vi "loadorsave_Option.vi"(6 "save?":bool, 8 "error in":errorcluster, 10 "Caldata in":T1={"分辨率"="", "Fps"=0, "工单号"="", "操作人"="", "增益模式"=enum."高低增益切换", "黑体设定温度1"=0.0, "温差范围1"=0.0, "出图到测温等待时间"=0.0, "调焦数值min"=0, "盲元阈值"=0.0, "盲元采样帧数"=0, "调焦数值min2"=0, "黑体设定温度2"=0.0, "温差范围2"=0.0, "ID选择"=enum."新ID", "快门时间间隔设置"={"快门第一次延时时间"=200, "快门第二次延时时间"=200, "切换增益后快门第一次延时时间"=200, "切换增益后快门第二次延时时间"=200}, "产品名"="Tiny1-C", "镜头"="02011X", "测温功能"="WR", "产品料号"="", "打印机VISA"="", "焦距选择"=enum."Radio Selection 1", "工位"="0001", "服务器保存地址"=path ""}, 11 "Path in":path) -> (0 "error out":errorcluster, 2 "Caldata out":T1={"分辨率"="", "Fps"=0, "工单号"="", "操作人"="", "增益模式"=enum."高低增益切换", "黑体设定温度1"=0.0, "温差范围1"=0.0, "出图到测温等待时间"=0.0, "调焦数值min"=0, "盲元阈值"=0.0, "盲元采样帧数"=0, "调焦数值min2"=0, "黑体设定温度2"=0.0, "温差范围2"=0.0, "ID选择"=enum."新ID", "快门时间间隔设置"={"快门第一次延时时间"=200, "快门第二次延时时间"=200, "切换增益后快门第一次延时时间"=200, "切换增益后快门第二次延时时间"=200}, "产品名"="Tiny1-C", "镜头"="02011X", "测温功能"="WR", "产品料号"="", "打印机VISA"="", "焦距选择"=enum."Radio Selection 1", "工位"="0001", "服务器保存地址"=path ""}, 3 "Path out":path)   [LabVIEW 2016]
uses:
  Ctl/Option.ctl
panel:
  out "Caldata ctl":T1={"分辨率"="", "Fps"=0, "工单号"="", "操作人"="", "增益模式"=enum."高低增益切换", "黑体设定温度1"=0.0, "温差范围1"=0.0, "出图到测温等待时间"=0.0, "调焦数值min"=0, "盲元阈值"=0.0, "盲元采样帧数"=0, "调焦数值min2"=0, "黑体设定温度2"=0.0, "温差范围2"=0.0, "ID选择"=enum."新ID", "快门时间间隔设置"={"快门第一次延时时间"=200, "快门第二次延时时间"=200, "切换增益后快门第一次延时时间"=200, "切换增益后快门第二次延时时间"=200}, "产品名"="Tiny1-C", "镜头"="02011X", "测温功能"="WR", "产品料号"="", "打印机VISA"="", "焦距选择"=enum."Radio Selection 1", "工位"="0001", "服务器保存地址"=path ""}
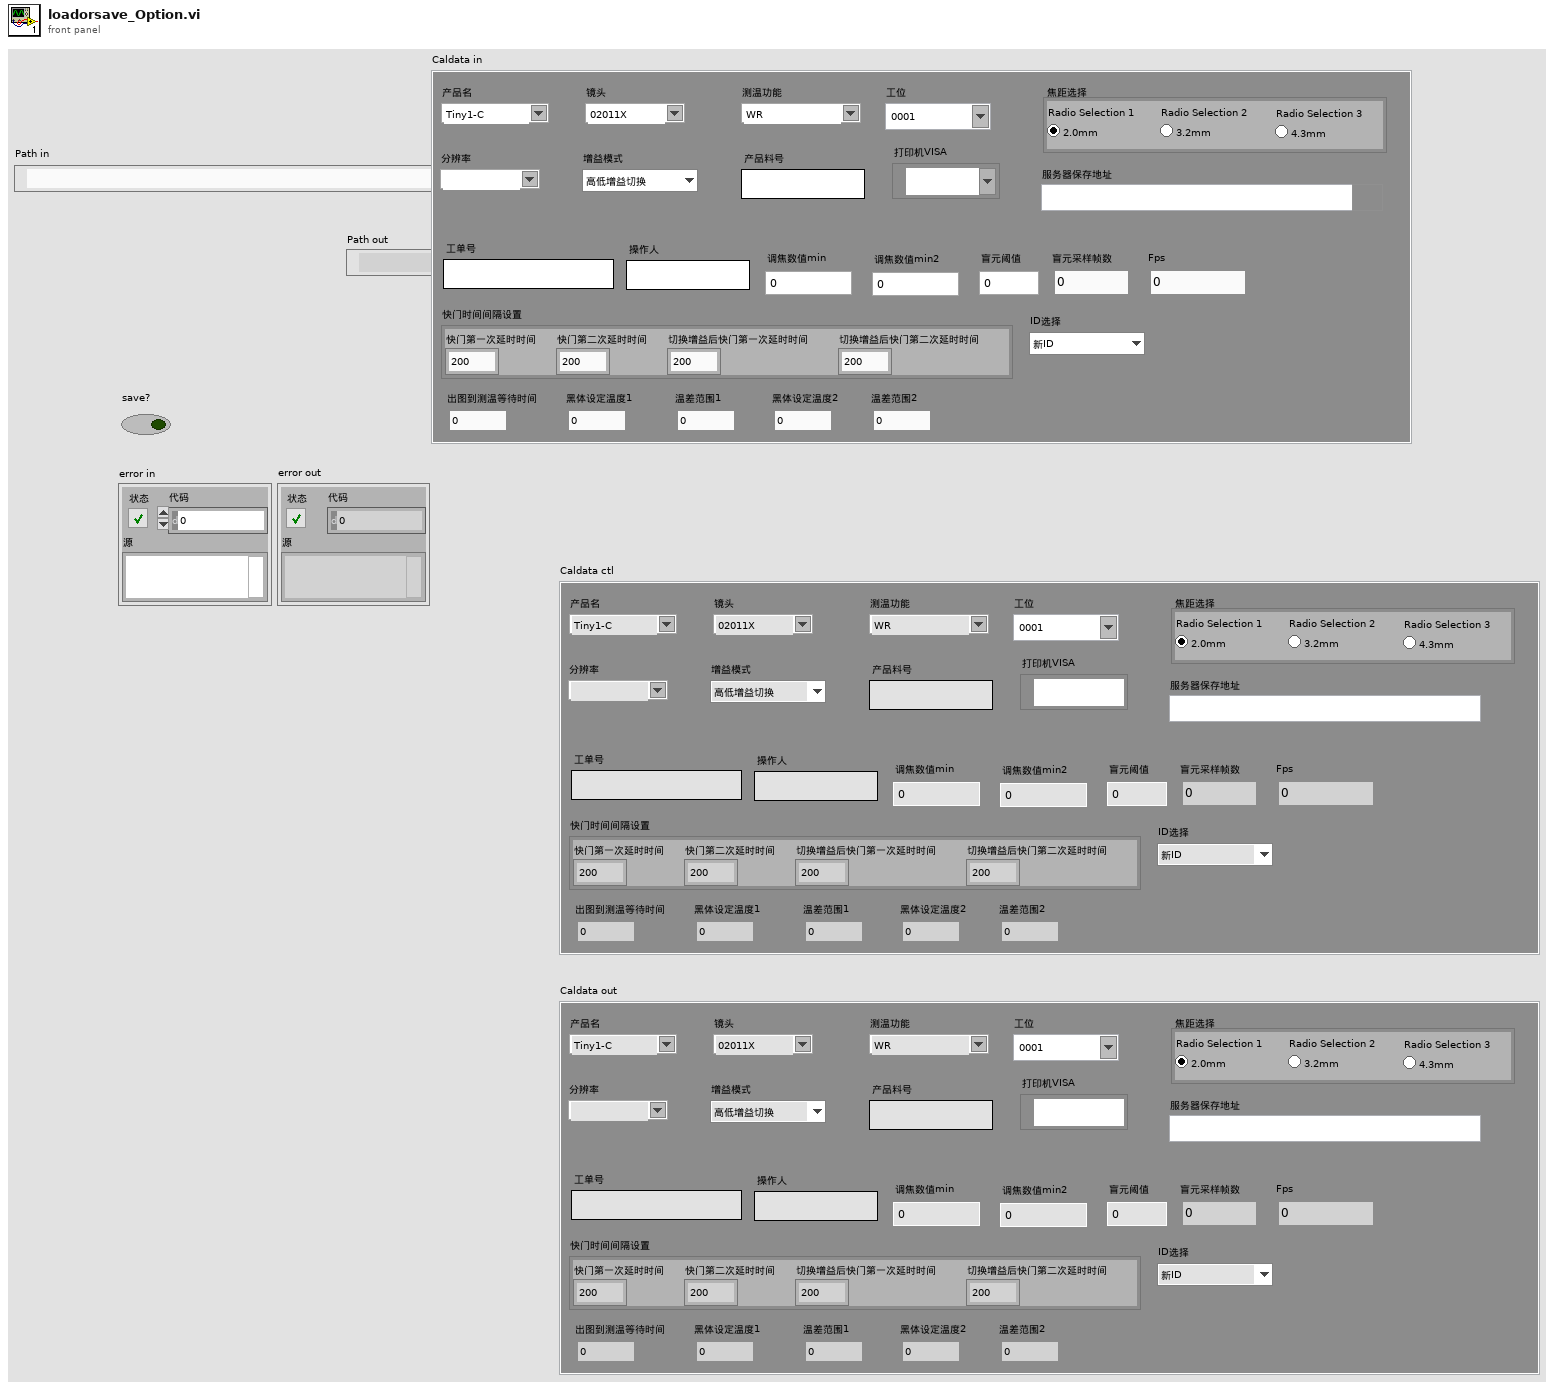
[diagram p1: front panel]
types:
  T1 = typedef "Option.ctl" = cluster{"分辨率":string, "Fps":u16, "工单号":string, "操作人":string, "增益模式":enum16{"高低增益切换", "高增益"}, "黑体设定温度1":dbl, "温差范围1":dbl, "出图到测温等待时间":dbl, "调焦数值min":i32, "盲元阈值":dbl, "盲元采样帧数":u16, "调焦数值min2":i32, "黑体设定温度2":dbl, "温差范围2":dbl, "ID选择":enum16{"旧ID", "新ID"}, "快门时间间隔设置":cluster{"快门第一次延时时间":u16, "快门第二次延时时间":u16, "切换增益后快门第一次延时时间":u16, "切换增益后快门第二次延时时间":u16}, "产品名":string, "镜头":string, "测温功能":string, "产品料号":string, "打印机VISA":refnum<visa-resource-name>, "焦距选择":enum32{"Radio Selection 1", "Radio Selection 2", "Radio Selection 3"}, "工位":string, "服务器保存地址":path}
  T2 = enum16{"open", "replace", "create", "open or create", "replace or create", "replace or create with confirmation"}
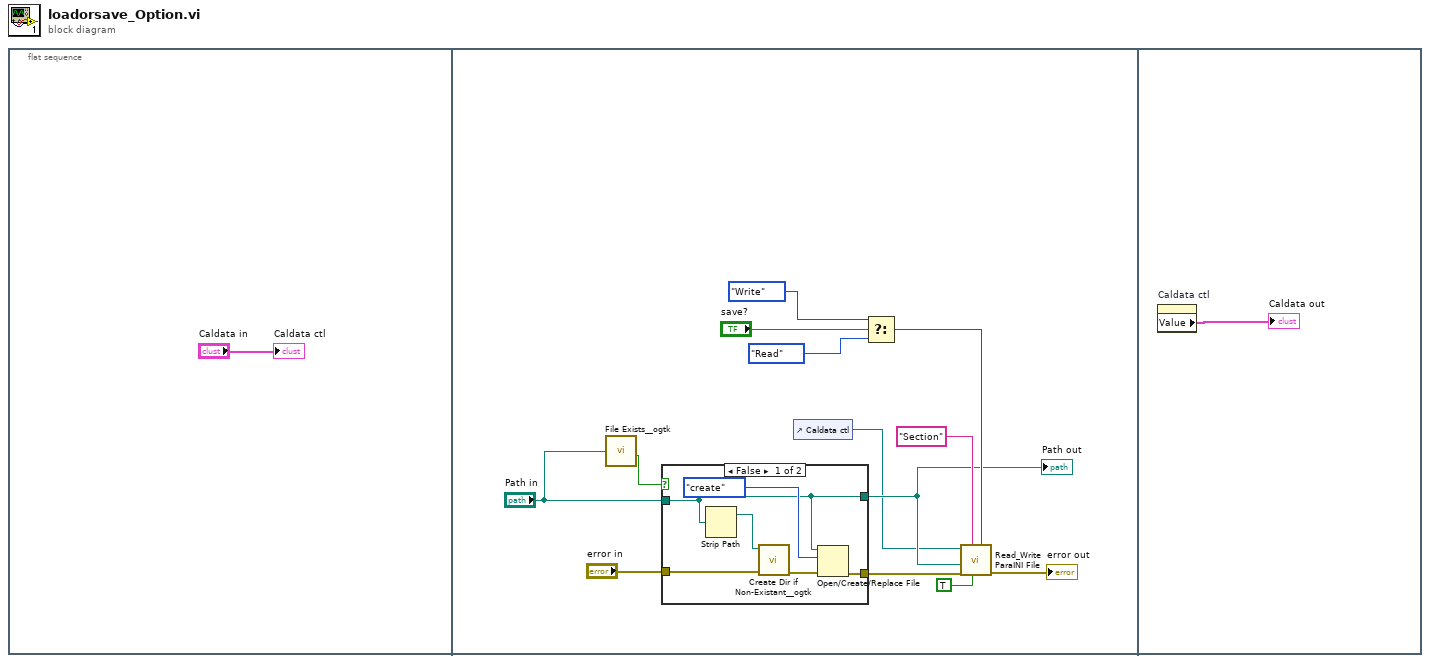
[diagram p0: block diagram]
diagram:
  n1 = flat-sequence {
    frame #0 {
      "Caldata ctl" <- "Caldata in"
    }
    frame #1 {
      n2 = call-poly "File Exists__ogtk.vi"("file path"="Path in") -> ("exists"=w9:bool)  [unwired: 6 in, 1 out]
      n3 = case shown="False" w9 {
        tunnel: "Path in" -> [w16 w22]
        tunnel: [w16 w22] -> w7
        tunnel: "error in" -> [w19 w21]
        tunnel: [w15 w21] -> w5
        frame False {
          n4 = Strip Path(path=w16) -> (stripped path=w20:path)  [unwired: 1 out]
          n5 = call "Create Dir if Non-Existant__ogtk.vi"("error in (no error)"=w19, "Directory Path"=w20) -> ("error out"=w18:errorcluster)  [unwired: 7 in, 2 out]
          n6 = Open/Create/Replace File(file path (use dialog)=w16, error in=w18, operation (0:open)=T2."create") -> (error out=w15:errorcluster)  [unwired: 3 in, 2 out]
        }
        frame True {
        }
      }
      "Path out" <- w7
      n7 = control-ref of="Caldata ctl"() -> (w3:refnum<vi>)
      n8 = Select(t=enum16{"Read", "Write"}."Write" ("Mode"), s="save?", f=enum16{"Read", "Write"}."Read" ("Mode")) -> (s? t:f=w11:enum16{"Read", "Write"})
      n9 = call "Read_Write ParaINI File.vi"("Mode"=w11, "Indicators too?"=TRUE, "Section"="Section", "error in"=w5, "Filepath"=w7, "Ctl Refnum"=w3) -> ("error out"=→"error out":errorcluster)  [unwired: 5 in]
    }
    frame #2 {
      n10 = property on="Caldata ctl" class="Clust (strict)"() -> ("Value"=→"Caldata out":T1)  [unwired: 2 in, 2 out]
    }
  }
